vi "AM Modulation Demo (Baseband-Sine) - Square - 副本.vi"() -> ()   [LabVIEW 2013]
uses:
  <vilib>/express/express analysis/Spectral/Block/exnSpectralBlock spectral measurements RMS poly.vi
  <vilib>/express/express analysis/Spectral/Block/exnSpectralBlock spectral measurements RMS DDT.vi
  <vilib>/express/express analysis/Spectral/Block/exnSpectralBlock spectral measurements power poly.vi
  <vilib>/express/express analysis/Spectral/Block/exnSpectralBlock spectral measurements power DDT.vi
  <vilib>/express/express analysis/Spectral/XNode/ExpressSpectralMeasurementsBlockNode.xnode
panel:
  in  "WAV Sample Rate":dbl=44100.0 caption="dt"
  in  "Mod. Freq.":dbl=2000.0 caption="Frequency"
  in  "LPF Cut-Off":dbl=10000.0 caption="Lower Cut-Off"
  in  "SNR (dB)":dbl(slide)=0.6 caption="Standard deviation" scale=-20.0..30.0
  out "Comparision":dynamicdata(graph)
  out "Baseband":dynamicdata(graph)
  out "DSB FFT":dynamicdata(graph)
  out "DSB sIGNAL":dynamicdata(graph)
  out "?":dbl=1.0
  in  "Carrier Amp.":dbl=1.0 caption="Amplitude"
  in  "stop":bool
  in  "Frequency Offset":dbl(slide)=1.0 scale=0.0..1000.0
  in  "Carrier Freq.":dbl=100000.0 caption="Frequency"
  out "DSB Squared":dynamicdata(graph)=[{"t0"=timestamp(0 s since 1904-01-01), "dt"=10.0, "Y"=array[50000 elements], "attributes"=variant("NI_ChannelName"=variant(string "Sine (Power Spectrum)"), "NI_ExpIsRelativeTime"=variant(bool TRUE), "NI_ExpStartTimeStamp"=variant(timestamp timestamp(3635665779.2842293 s since 1904-01-01)), "NI_ExpTimeStamp"=variant(timestamp timestamp(3635665779.2842293 s since 1904-01-01)), "NI_ExpXDimension"=variant(string "f"), "NI_OriginalChannelName"=variant(string "Sine"))}]
  # "Amplitude Modulation"
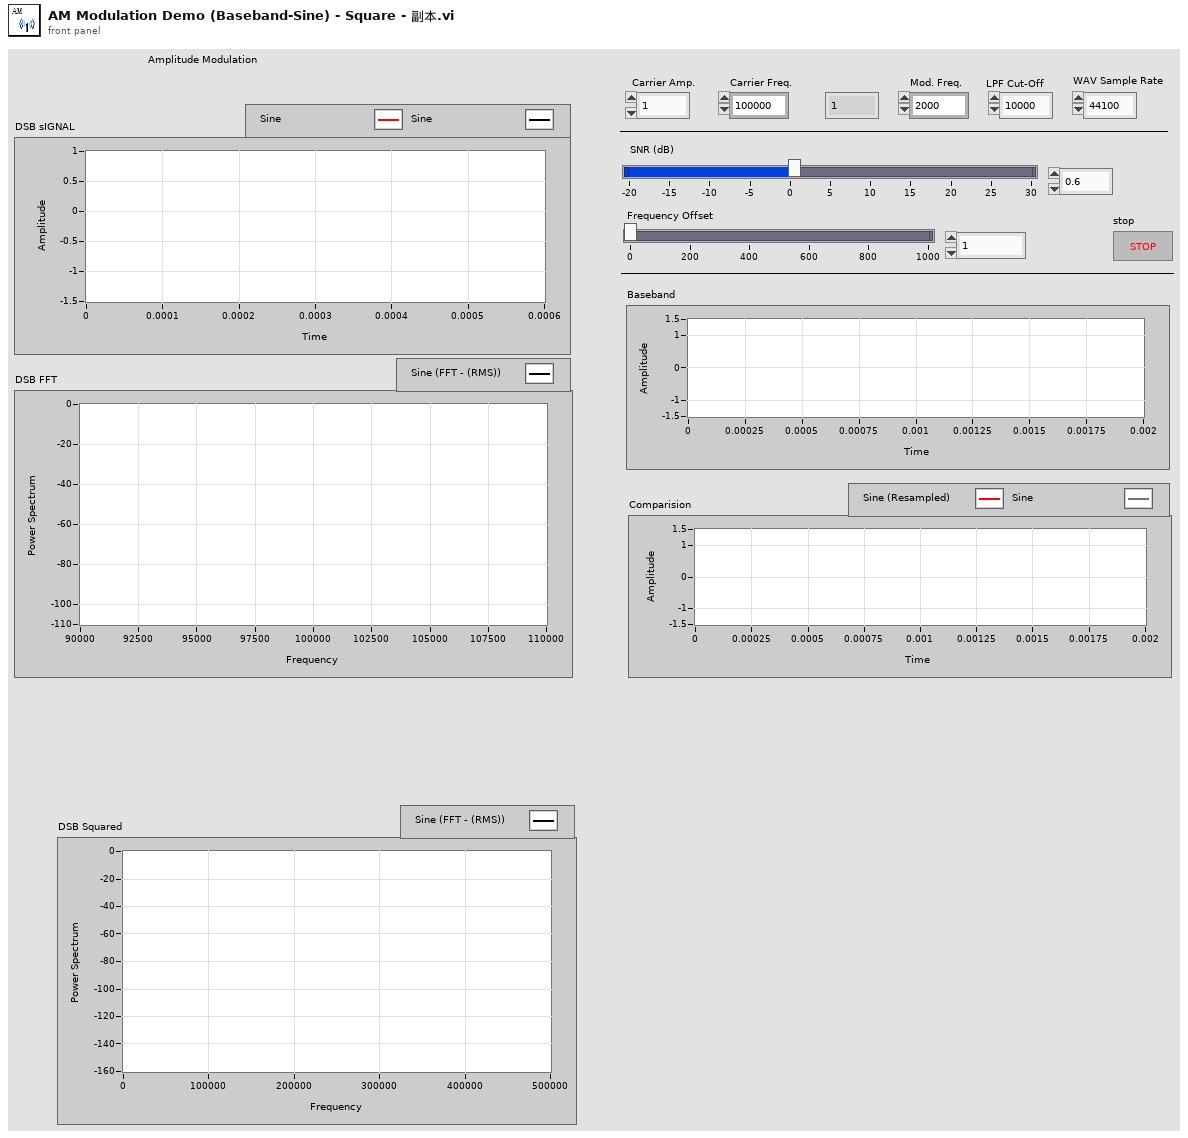
[diagram p1: front panel]
types:
  T1 = cluster{"averaging mode":u16, "weighting mode":u16, "number of averages":u32}
  T2 = cluster{"dB On (F)":bool, "unwrap phase (F)":bool, "convert to degree (F)":bool}
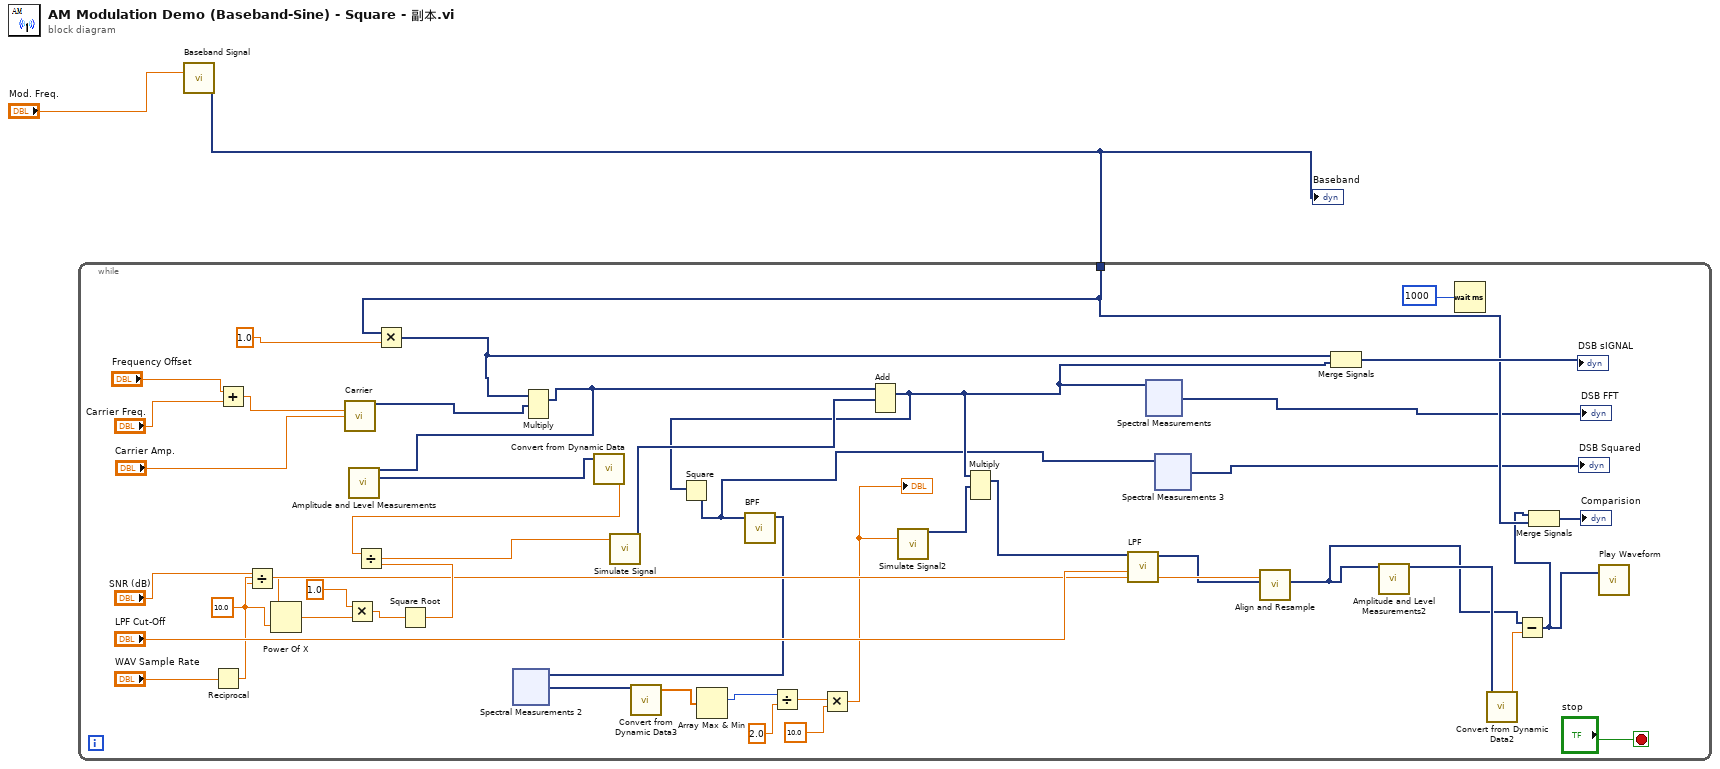
[diagram p0: block diagram]
diagram:
  n1 = call "Baseband Signal"("Frequency"="Mod. Freq.") -> ("Sine"=w1:dynamicdata)  [unwired: 13 in, 1 out]
  "Baseband" <- w1
  n2 = while {
    tunnel: w1 -> [w30]
    stop <- "stop" stop-if-true
    w26 = 10.0
    n3 = Reciprocal(x="WAV Sample Rate") -> (1/x=w34:dbl)
    n4 = Add(x="Frequency Offset", y="Carrier Freq.") -> (x+y=w19:dbl)
    n5 = Divide(x="SNR (dB)", y=w26) -> (x/y=w27:dbl)
    n6 = Power Of X(1:w26, 2:w27) -> (0:w25:dbl)
    n7 = call "Carrier"("Frequency"=w19, "Amplitude"="Carrier Amp.") -> ("Sine"=w46:dynamicdata)  [unwired: 12 in, 1 out]
    n8 = Multiply(x=1.0, y=w25) -> (x*y=w40:dbl)
    n9 = Multiply(x=w30, y=1.0) -> (x*y=w20:dynamicdata)
    n10 = Square Root(x=w40) -> (sqrt(x)=w38:dbl)
    n11 = Multiply(1:w46, 2:w20) -> (0:w37:dynamicdata)  [unwired: 1 in, 1 out]
    n12 = call "Amplitude and Level Measurements"("Signals"=w37) -> ("RMS"=w44:dynamicdata)  [unwired: 13 in, 1 out]
    n13 = call "Convert from Dynamic Data"("Dynamic Data Type"=w44) -> ("Scalar"=w39:dbl)  [unwired: 3 in]
    n14 = Divide(x=w39, y=w38) -> (x/y=w24:dbl)
    n15 = call "Simulate Signal"("Standard deviation"=w24) -> ("DC with Gaussian Noise"=w36:dynamicdata)  [unwired: 13 in, 1 out]
    n16 = Add(1:w36, 2:w37) -> (0:w13:dynamicdata)  [unwired: 1 in, 1 out]
    n17 = Square(x=w13) -> (x^2=w4:dynamicdata)
    n18 = call "BPF"("Signal"=w4) -> ("Filtered Signal"=w12:dynamicdata)  [unwired: 9 in, 1 out]
    n19 = xnode "Spectral Measurements 2"("Signals"=w12) -> ("Power Spectrum"=w11:dynamicdata)  [unwired: 1 in, 1 out]
    n20 = call "Convert from Dynamic Data3"("Dynamic Data Type"=w11) -> ("Array"=w10:dbl[])  [unwired: 3 in]
    n21 = Array Max & Min(array=w10) -> (max index (indices)=w9:i32)  [unwired: 3 out]
    n22 = Divide(x=w9, y=2.0) -> (x/y=w7:dbl)
    n23 = Multiply(x=w7, y=10.0) -> (x*y=w5:dbl)
    "?" <- w5
    n24 = call "Simulate Signal2"("Frequency"=w5) -> ("Sine"=w18:dynamicdata)  [unwired: 13 in, 1 out]
    n25 = Multiply(1:w18, 2:w13) -> (0:w17:dynamicdata)  [unwired: 1 in, 1 out]
    n26 = call "LPF"("Lower Cut-Off"="LPF Cut-Off", "Signal"=w17) -> ("Filtered Signal"=w33:dynamicdata)  [unwired: 8 in, 1 out]
    n27 = xnode "Spectral Measurements"("Signals"=w13) -> ("FFT - (RMS)"=→"DSB FFT":dynamicdata)  [unwired: 1 in, 2 out]
    n28 = xnode "Spectral Measurements 3"("Signals"=w4) -> ("FFT - (RMS)"=→"DSB Squared":dynamicdata)  [unwired: 1 in, 2 out]
    n29 = call "Align and Resample"("dt"=w34, "Signals"=w33) -> ("Resampled Signals"=w21:dynamicdata)  [unwired: 7 in, 2 out]
    n30 = Merge Signals(w20, w13) -> (→"DSB sIGNAL":dynamicdata)
    n31 = call "Amplitude and Level Measurements2"("Signals"=w21) -> ("Mean (DC)"=w22:dynamicdata)  [unwired: 13 in, 1 out]
    n32 = Wait (ms)(milliseconds to wait=1000) -> ()  [unwired: 1 out]
    n33 = call "Convert from Dynamic Data2"("Dynamic Data Type"=w22) -> ("Scalar"=w29:dbl)  [unwired: 3 in]
    n34 = Subtract(x=w21, y=w29) -> (x-y=w23:dynamicdata)
    n35 = Merge Signals(w23, w30) -> (→"Comparision":dynamicdata)
    n36 = call "Play Waveform"("Data"=w23) -> ()  [unwired: 18 in, 1 out]
  }
